vi "IV_analysis_tdms_Erin.vi"() -> ()   [LabVIEW 2019]
uses:
  <userlib>/Levylab/LV to ITX/LVtoITX.lvclass
panel:
  out "IV":cluster{dbl[], dbl[]}[](graph)
  out "Conductance":cluster{dbl[], dbl[]}[](graph)
  in  "average length":i32=300
  in  "dv":dbl=300.0 format="%#_13g"
  out "?":dbl[][](graph)
  out "?":dbl[][](graph)
  out "?":dbl[][](graph)
  out "?":dbl[][](graph)
  in  "X Step":dbl=1e-06 format="%#_6p"
  in  "X High":dbl=0.003 format="%#_6p"
  in  "X Low":dbl=-0.003 format="%#_6p"
  in  "# per group":i32=1
  in  "Group #":i32=801
  in  "File or Folder Path 2":path=path "G:/My Drive/ansom/Data/PPMSDAQ/2020/PPMS 1/SA02821O.20201201/04-Biasspectr-IV"
  in  "LV to itx":T1={"A"=10, "B"=4, "C"=5, "D"=5, "E"=2, "N1"=3, "N2"=2, "N3"=0, "N4"=0}
  in  "index in group":i32
  in  "offset":i32=1
  in  "LV/ITX?":bool=TRUE
  # "Current"
  # "V4T+"
  # "V4T-"
  # "Drive current"
  # "Vbg/Vsg"
  # "Temp/B"
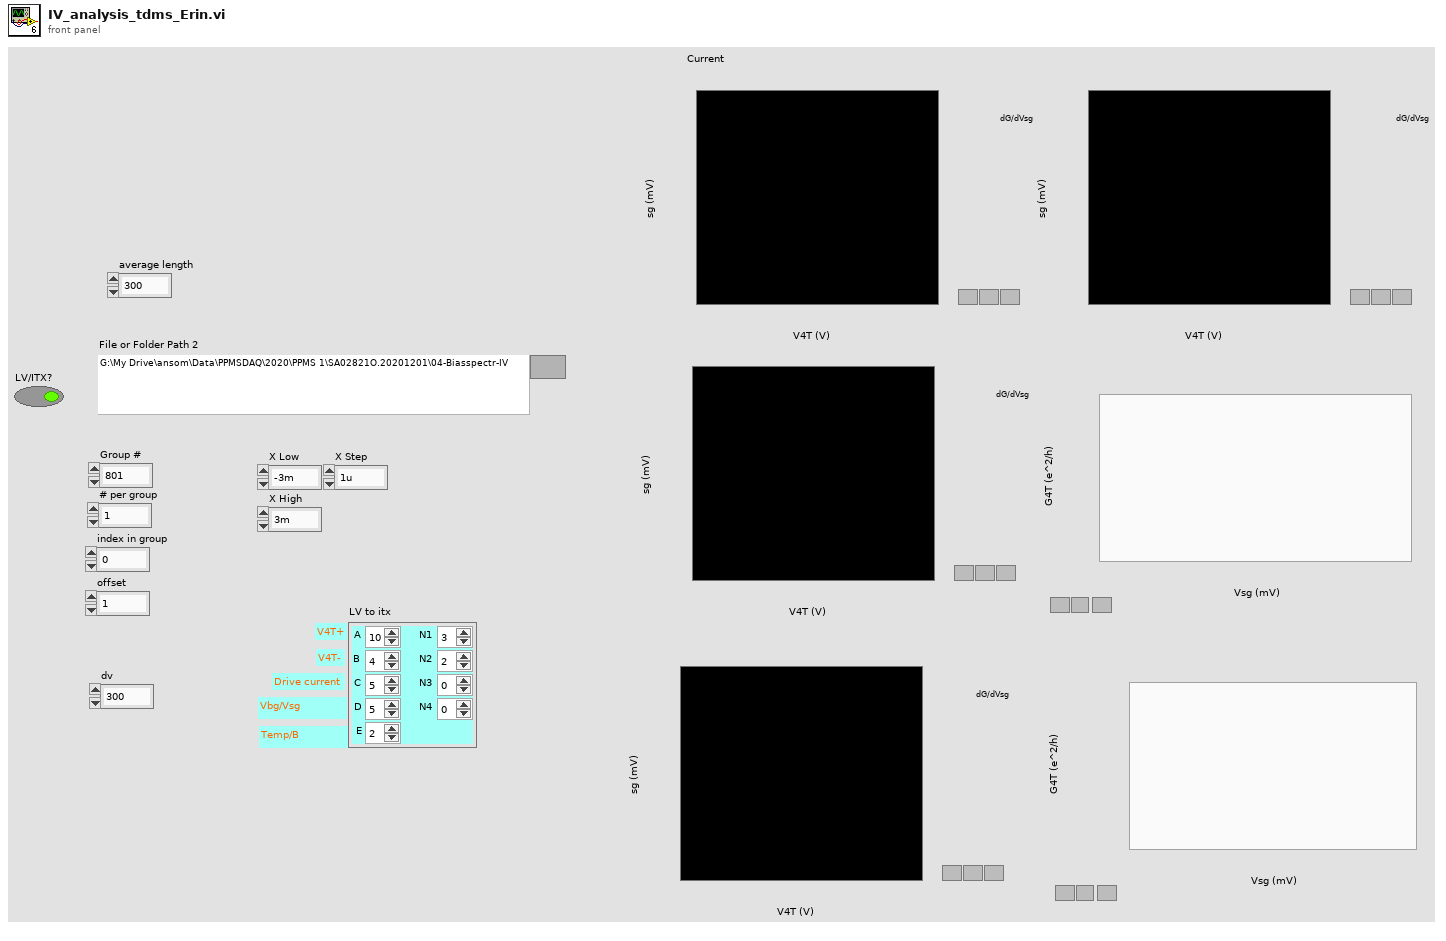
[diagram p1: front panel]
types:
  T1 = cluster{"A":i32, "B":i32, "C":i32, "D":i32, "E":i32, "N1":i32, "N2":i32, "N3":i32, "N4":i32}
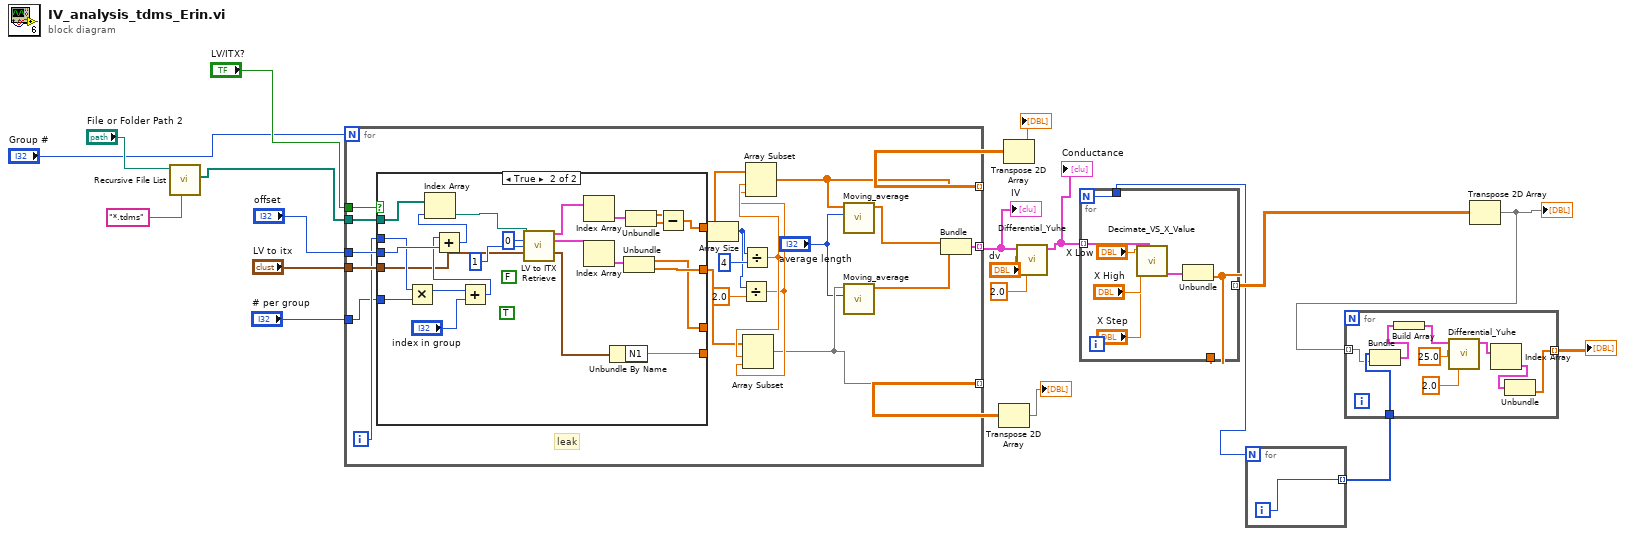
[diagram p0: block diagram]
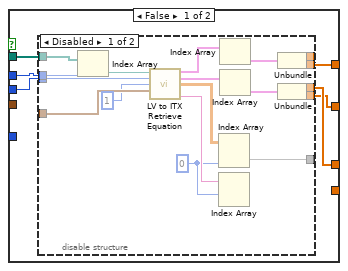
[diagram p2: hidden frame]
diagram:
  n1 = call <vilib>:"Recursive File List.vi"("pattern"="*.tdms", "Folder Path"="File or Folder Path 2") -> ("All Files in Dir"=w18:path[])  [unwired: 5 in, 4 out]
  n2 = for {
    N: "Group #" -> [_]
    tunnel: w18 -> [w40]
    tunnel: "LV to itx" -> [w39]
    tunnel: "offset" -> [w38]
    tunnel: "LV/ITX?" -> [w37]
    tunnel: "# per group" -> [w35]
    tunnel: [w34] -> w2 mode=indexing
    tunnel: [w26] -> w7 mode=indexing
    tunnel: [w23] -> w5 mode=indexing
    i -> [w36]
    # "leak"
    n3 = case shown="True" w37 {
      tunnel: w40 -> [w42 w87]
      tunnel: w39 -> [_ w79]
      tunnel: [w45 w73] -> _
      tunnel: [w44 w74] -> w28
      tunnel: [_ w88] -> _
      tunnel: [w46 w68] -> w29
      tunnel: w38 -> [w43 w86]
      tunnel: w36 -> [w41 w85]
      tunnel: w35 -> [_ w84]
      frame False {
        n4 = disable-structure shown="Disabled" {
          disable-tunnel: _ -> [w65 _]
          disable-tunnel: [w58 _] -> _
          disable-tunnel: [w57 _] -> w46
          disable-tunnel: [w56 _] -> w45
          disable-tunnel: [w55 _] -> w44
          disable-tunnel: [w54 _] -> _
          disable-tunnel: w43 -> [w53 _]
          disable-tunnel: w42 -> [w49 _]
          disable-tunnel: w41 -> [w48 _]
          frame Disabled {
            w50 = 0 ("length")
            n5 = Index Array(array=w49, index=w48) -> (element=w47:path)
            n6 = call <userlib>:"LV to ITX  Retrieve Equation.vi"("File or Folder Path"=w47, "offset"=w53, "length"=1, "index"=w65) -> ("y1 vs g"=w63:cluster{dbl[], dbl[]}[], "y2 vs g"=w61:cluster{dbl[], dbl[]}[], "2D"=w59:dbl[][], "Comments"=w52:string)  [unwired: 7 in, 1 out]
            n7 = Index Array(array=w59, index (col)=w50) -> (element=w54:dbl[])  [unwired: 1 in]
            n8 = Index Array(array=w52, index (row)=w50) -> (element=w51)  [unwired: 1 in]
            n9 = Index Array(array=w63) -> (element=w62:cluster{dbl[], dbl[]})  [unwired: 1 in]
            n10 = Index Array(array=w61) -> (element=w60:cluster{dbl[], dbl[]})  [unwired: 1 in]
            n11 = Unbundle(w62) -> (w58:dbl[], w57:dbl[])
            n12 = Unbundle(w60) -> (w56:dbl[], w55:dbl[])
          }
          frame Enabled {
          }
        }
      }
      frame True {
        (unwired) FALSE ("file contains 2D data?")
        (unwired) TRUE ("stop")
        n13 = Multiply(x=w85, y=w84) -> (x*y=w83:i32)
        n14 = Add(x=w83, y="index in group") -> (x+y=w81:i32)
        n15 = Add(x=w81, y=w86) -> (x+y=w67:i32)
        n16 = Index Array(array=w87, index=w67) -> (element=w78:path)
        n17 = call <userlib>:"LV to ITX  Retrieve.vi"("File or Folder Path"=w78, "offset"=0, "length"=1, "index"=w79) -> ("A vs B"=w72:cluster{dbl[], dbl[]}[], "C vs D"=w76:cluster{dbl[], dbl[]}[], "N"=w77:cluster{"N1":dbl, "N2":dbl, "N3":dbl, "N4":dbl})  [unwired: 7 in, 2 out]
        n18 = Index Array(array=w72) -> (element=w71:cluster{dbl[], dbl[]})  [unwired: 1 in]
        n19 = Index Array(array=w76) -> (element=w75:cluster{dbl[], dbl[]})  [unwired: 1 in]
        n20 = Unbundle By Name(w77) -> ("N1"=w88:dbl)
        n21 = Unbundle(w75) -> (w73:dbl[], w74:dbl[])
        n22 = Unbundle(w71) -> (w69:dbl[], w70:dbl[])
        n23 = Subtract(x=w70, y=w69) -> (x-y=w68:dbl[])
      }
    }
    n24 = Array Size(array=w29) -> (size(s)=w31:i32)
    n25 = Divide(x=w31, y=2.0) -> (x/y=w27:dbl)
    n26 = Divide(x=w31, y=4) -> (x/y=w30:dbl)
    n27 = Array Subset(array=w28, index=w30, length=w27) -> (w26:dbl[])
    n28 = Array Subset(array=w29, index=w30, length=w27) -> (w23:dbl[])
    n29 = call "Moving_average.vi"("average length"="average length", "Input"=w23) -> ("Output"=w24:dbl[])  [unwired: 9 in]
    n30 = call "Moving_average.vi"("average length"="average length", "Input"=w26) -> ("Output"=w25:dbl[])  [unwired: 9 in]
    n31 = Bundle("Output"=w24, "Output"=w25) -> (w34:cluster{"Output":dbl[], "Output":dbl[]})  [unwired: 1 in]
  }
  "IV" <- w2
  n32 = Transpose 2D Array(2D array=w7) -> (transposed array=→"?":dbl[][])
  n33 = Transpose 2D Array(2D array=w5) -> (transposed array=→"?":dbl[][])
  n34 = call "Differential_Yuhe.vi"("step"=2.0, "dv"="dv", "A vs B"=w2) -> ("A vs B 2"=w3:cluster{dbl[], dbl[]}[])  [unwired: 8 in]
  "Conductance" <- w3
  n35 = for {
    N -> [w89]
    tunnel: w3 -> [w95] mode=indexing
    tunnel: [w90] -> w11 mode=indexing
    tunnel: [w90] -> _
    tunnel: [w89] -> w9
    n36 = call "Decimate_VS_X_Value.vi"("XY Graph kind 1"=w95, "X Step"="X Step", "X High"="X High", "X Low"="X Low") -> ("Interpreted"=w91:cluster{dbl[], dbl[]})  [unwired: 6 in, 1 out]
    n37 = Unbundle(w91) -> (w90:dbl[])  [unwired: 1 out]
  }
  n38 = for {
    N: w9 -> [_]
    tunnel: [w96] -> w10 mode=indexing
    i -> [w96]
  }
  n39 = Transpose 2D Array(2D array=w11) -> (transposed array=w8:dbl[][])
  "?" <- w8
  n40 = for {
    tunnel: w8 -> [w102] mode=indexing
    tunnel: w10 -> [w103]
    tunnel: [w97] -> w1 mode=indexing
    n41 = Bundle(w103, w102) -> (w101:cluster{i32[], dbl[]})  [unwired: 1 in]
    n42 = Build Array(w101) -> (w100:cluster{i32[], dbl[]}[])
    n43 = call "Differential_Yuhe.vi"("step"=2.0, "dv"=25.0, "A vs B"=w100) -> ("A vs B 2"=w99:cluster{dbl[], dbl[]}[])  [unwired: 8 in]
    n44 = Index Array(array=w99) -> (element=w98:cluster{dbl[], dbl[]})  [unwired: 1 in]
    n45 = Unbundle(w98) -> (w97:dbl[])  [unwired: 1 out]
  }
  "?" <- w1
